vi "To ASCII.vi"(0 "Experiment State":T1={"error"={"status"=FALSE, "code"=0, "source"=""}, "Digitizer DAQmx Tasks"={"TaskArray"=[]}, "Digitizer Settings"={"Channel Settings"=[], "Card Settings"=[]}, "Synchronization Settings"={"Synchronizer"="PXI1Slot2", "source terminal"="GlobalSoftwareTrigger"}, "Digitizer Data"=[], "Next Shot#"="0", "System Message"="", "User Shot Notes"="", "Timing Settings"={"Timing Card Settings"=[], "Timing Channel Settings"=[[{"Delay (s)"=2.559999942779541, "Pulse width (s)"=0.009999999776482582, "Active"=TRUE, "Channel Name"="Fiber 8", "counter"="PXI1Slot8/ctr7", "FrontPanelTime"=2.559999942779541}]]}, "Timing Tasks"={"TaskArray"=[]}, "Tree"="0", "Time Card/Channels"=[2, 8], "DAQ Card/Channels"=[3, 8]} {"Timing Settings"."Timing Channel Settings"."FrontPanelTime" format="%.3p"; "Timing Settings"."Timing Channel Settings"."Pulse width (s)" format="%.3p"; "Timing Settings"."Timing Channel Settings"."Delay (s)" format="%.3p"; "Digitizer Settings"."Card Settings"."Global Edge Type" items=["Rising"=10280, "Falling"=10171]; "Digitizer Settings"."Card Settings"."Sample Rate" format="%#_3p"}) -> ()   [LabVIEW 2013]
uses:
  Controls/ExperimentStateCluster.ctl
  Controls/DigitizerSettingsChannelSettings.ctl
  Controls/DigitizerSettingsCardSettingsArray.ctl
  Controls/DigitizerSettingsCardSettings.ctl
  Controls/TimingSettings.ctl
  Controls/TimingCardSettings.ctl
  Controls/TimingChannelSettings.ctl
  <vilib>/Utility/file.llb/Write To Spreadsheet File (string).vi
  <vilib>/Waveform/WDTFileIO.llb/Export Waveforms To Spreadsheet File (1D).vi
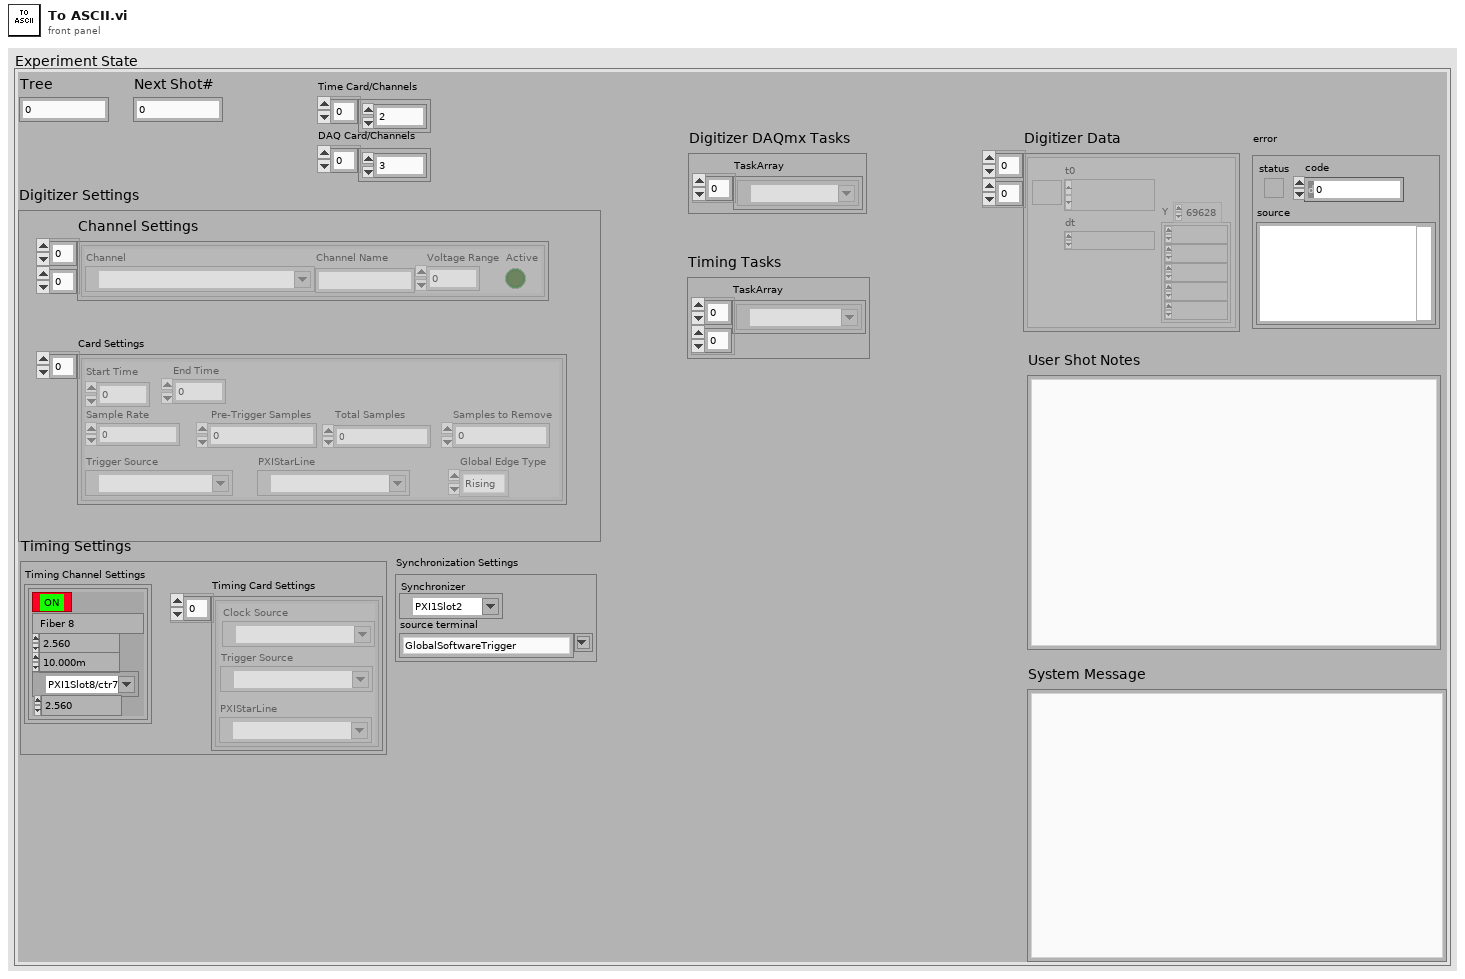
[diagram p1: front panel]
types:
  T1 = typedef "ExperimentStateCluster.ctl" = cluster{"error":errorcluster, "Digitizer DAQmx Tasks":cluster{"TaskArray":refnum<k21>[]}, "Digitizer Settings":cluster{"Channel Settings":T2[][], "Card Settings":T3}, "Synchronization Settings":cluster{"Synchronizer":refnum<k15>, "source terminal":string}, "Digitizer Data":waveform(dbl)[][], "Next Shot#":string, "System Message":string, "User Shot Notes":string, "Timing Settings":T5, "Timing Tasks":cluster{"TaskArray":refnum<k21>[][]}, "Tree":string, "Time Card/Channels":i32[], "DAQ Card/Channels":i32[]}
  T2 = typedef "DigitizerSettingsChannelSettings.ctl" = cluster{"Channel":tag, "Channel Name":string, "Voltage Range":dbl, "Active":bool}
  T3 = typedef "DigitizerSettingsCardSettingsArray.ctl" = T4[]
  T4 = typedef "DigitizerSettingsCardSettings.ctl" = cluster{"Start Time":dbl, "End Time":dbl, "Sample Rate":dbl, " Pre-Trigger Samples":u32, "Total Samples":i32, "Samples to Remove":u32, "Trigger Source":tag, "Global Edge Type":i32, "PXIStarLine":tag}
  T5 = typedef "TimingSettings.ctl" = cluster{"Timing Card Settings":T6[], "Timing Channel Settings":T7[][]}
  T6 = typedef "TimingCardSettings.ctl" = cluster{"Trigger Source":tag, "Clock Source":tag, "PXIStarLine":tag}
  T7 = typedef "TimingChannelSettings.ctl" = cluster{"Delay (s)":dbl, "Pulse width (s)":dbl, "Active":bool, "Channel Name":string, "counter":tag, "FrontPanelTime":dbl}
  T8 = cluster{"Channel Settings":T2[][], "Card Settings":T3}
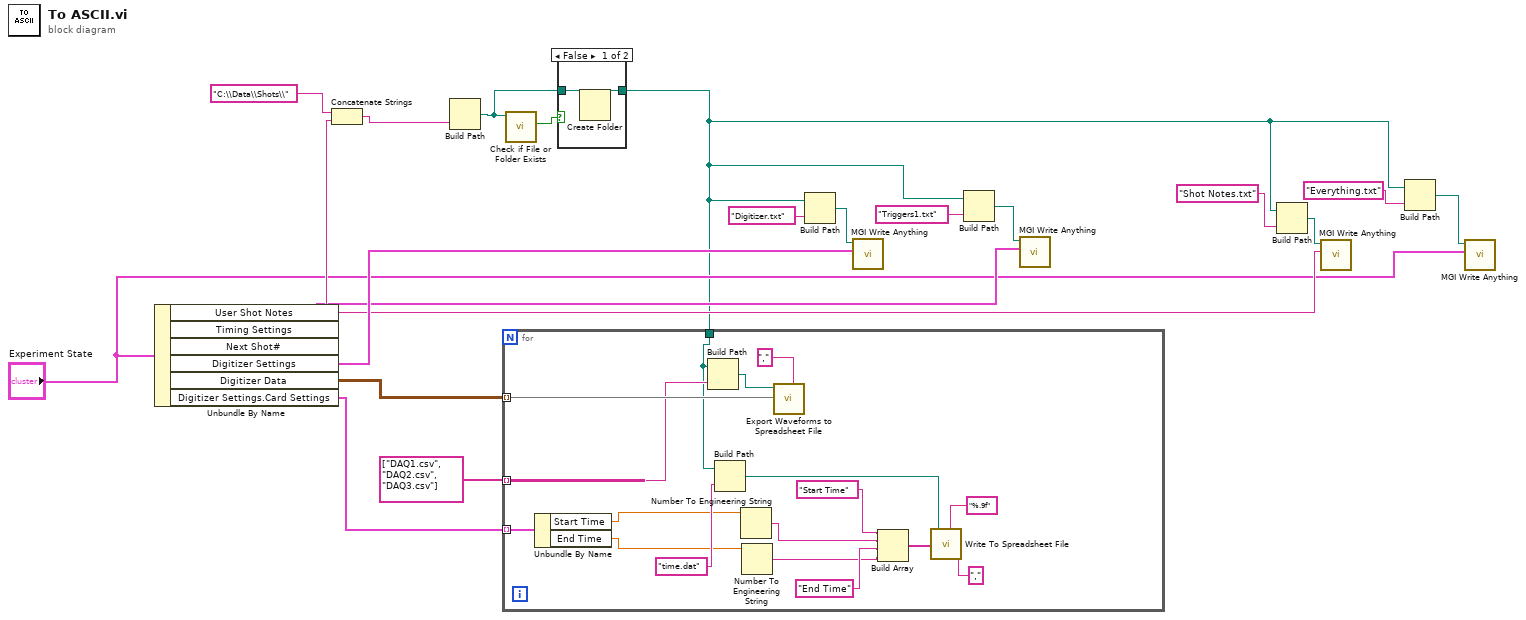
[diagram p0: block diagram]
diagram:
  n1 = Unbundle By Name("Experiment State") -> ("User Shot Notes"=w7:string, "Timing Settings"=w13:T5, "Next Shot#"=w21:string, "Digitizer Settings"=w14:T8, "Digitizer Data"=w18:waveform(dbl)[][], "Digitizer Settings.Card Settings"=w1:T3)
  n2 = Concatenate Strings("C:\\Data\\Shots\\" ("name or relative path"), w21) -> (w19:string)
  n3 = Build Path(name or relative path=w19) -> (appended path=w16:path)  [unwired: 1 in]
  n4 = call <vilib>:"Check if File or Folder Exists.vi"("path"=w16) -> ("file or folder exists?"=w15:bool)  [unwired: 8 in, 2 out]
  n5 = case shown="False" w15 {
    tunnel: [w22 w24] -> w4
    tunnel: w16 -> [w23 w24]
    frame False {
      n6 = Create Folder(path (use dialog)=w23) -> (created path=w22:path)  [unwired: 2 in, 2 out]
    }
    frame True {
    }
  }
  n7 = for {
    tunnel: w18 -> [w40] mode=indexing
    tunnel: w4 -> [w37]
    tunnel: string[] ["DAQ1.csv", "DAQ2.csv", "DAQ3.csv"] -> [w39] mode=indexing
    tunnel: w1 -> [w27] mode=indexing
    n8 = Unbundle By Name(w27) -> ("Start Time"=w26:dbl, "End Time"=w25:dbl)
    n9 = Build Path(base path=w37, name or relative path=w39) -> (appended path=w41:path)
    n10 = Build Path(base path=w37, name or relative path="time.dat") -> (appended path=w35:path)
    n11 = Number To Engineering String(4:w26) -> (0:w33:string)  [unwired: 3 in]
    n12 = Number To Engineering String(4:w25) -> (0:w31:string)  [unwired: 3 in]
    n13 = call-poly <vilib>:"Export Waveforms to Spreadsheet File.vi"("delimiter (Tab)"=",", "waveforms"=w40, "file path (dialog if empty)"=w41) -> ()  [unwired: 7 in, 2 out]
    n14 = Build Array("Start Time" ("string"), w33, "End Time" ("string"), w31) -> (w30:string[])
    n15 = call-poly <vilib>:"Write To Spreadsheet File.vi"("delimiter (\\t)"="," ("delimiter (\\t)"), "format (%s)"="%.9f", "1D data"=w30, "file path (dialog if empty)"=w35) -> ()  [unwired: 4 in, 1 out]
  }
  n16 = Build Path(base path=w4, name or relative path="Digitizer.txt") -> (appended path=w11:path)
  n17 = call <userlib>:"MGI Write Anything.vi"("Anything"=w14, "Path (dialog)"=w11) -> ()  [unwired: 7 in, 3 out]
  n18 = Build Path(base path=w4, name or relative path="Triggers1.txt") -> (appended path=w9:path)
  n19 = call <userlib>:"MGI Write Anything.vi"("Anything"=w13, "Path (dialog)"=w9) -> ()  [unwired: 7 in, 3 out]
  n20 = Build Path(base path=w4, name or relative path="Shot Notes.txt") -> (appended path=w8:path)
  n21 = call <userlib>:"MGI Write Anything.vi"("Anything"=w7, "Path (dialog)"=w8) -> ()  [unwired: 7 in, 3 out]
  n22 = Build Path(base path=w4, name or relative path="Everything.txt") -> (appended path=w3:path)
  n23 = call <userlib>:"MGI Write Anything.vi"("Anything"="Experiment State", "Path (dialog)"=w3) -> ()  [unwired: 7 in, 3 out]
